vi "TRAJECTORY_CREATE_QUINTIC_BEGIN.vi"() -> (0 "Trajectory \ncalculation \nerror":errorcluster, 2 "Trajectory Items":i32, 3 "TotalTImeSecs":dbl)   [LabVIEW 2019]
uses:
  <vilib>/Rock Robotics/WPI/ThirdParty/JAS_Junk/TrajLib/Rotation_CreateAngle.vi
  <vilib>/Rock Robotics/WPI/ThirdParty/JAS_Junk/TrajLib/Translation_Create.vi
  <vilib>/Rock Robotics/SystemInterfaces/NetworkCommunication/NetComm_UsageReport_report.vi
  <vilib>/Rock Robotics/WPI/ThirdParty/JAS_Junk/TrajLib/DiffDriveKinematicsConstraint_New.vi
  <vilib>/Rock Robotics/WPI/ThirdParty/JAS_Junk/TrajLib/CentripetalAccelConstraint_New.vi
  <vilib>/Rock Robotics/WPI/ThirdParty/JAS_Junk/TrajLib/Util_LibraryGlobals.vi
  <vilib>/Rock Robotics/WPI/ThirdParty/JAS_Junk/TrajLib/Trajectory_Library.lvlib
panel:
  in  "WayPoints":T1(array[cluster])=[{"X Inches"=15.0, "Y Inches"=105.0, "Heading\nDegrees"=-45.0}, {"X Inches"=105.0, "Y Inches"=65.0, "Heading\nDegrees"=0.0}, {"X Inches"=210.0, "Y Inches"=105.0, "Heading\nDegrees"=45.0}]
  in  "Use Diff Drive\nKinematic\nConstraint":bool=TRUE
  in  "Use Centripetal\nAcceleration\nConstaint":bool=TRUE
  out "Wheelbase Width":dbl=0.66 format="%20.4f"
  out "MaxAcceleration":dbl=1.3 format="%17.4f"
  out "MaxVelocity":dbl=2.0 format="%17.4f"
  out "Max Cent Accel":dbl=1.0 format="%20.4f"
  in  "Max Cent Accel INCHES/SEC^2":dbl=15.0 format="%20.1f"
  in  "MaxAcceleration INCHES/SEC^2":dbl=30.0 format="%17.1f"
  in  "MaxVelocity Fraction":dbl=0.666 format="%17.3f"
  # "TRAJECTORY CONFIGURATION"
  # "20.9 real"
  # "TRAJECTORY DEFINITION"
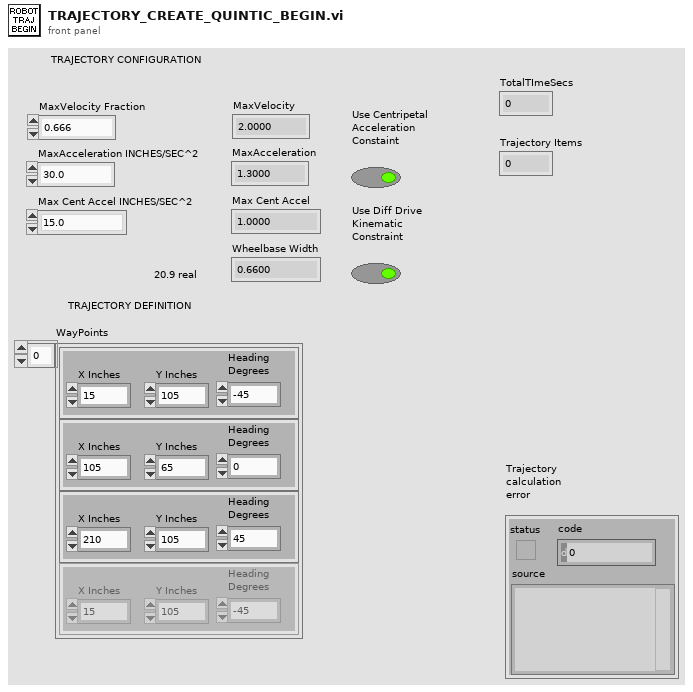
[diagram p1: front panel]
types:
  T1 = cluster{"X Inches":dbl, "Y Inches":dbl, "Heading\nDegrees":dbl}[]
  T2 = typedef "Trajectory_Library.lvlib/POSE2D.ctl" = cluster{"TRANSLATION":T3, "ROTATION":T4}
  T3 = typedef "Trajectory_Library.lvlib/TRANSLATION2D.ctl" = cluster{"X":dbl, "Y":dbl}
  T4 = typedef "Trajectory_Library.lvlib/ROTATION2D.ctl" = cluster{"VALUE":dbl, "COS":dbl, "SIN":dbl}
  T5 = typedef "Trajectory_Library.lvlib/TRAJ_CONFIG.ctl" = cluster{"MaxVelocity":dbl, "Max Acceleration":dbl, "StartVelocity":dbl, "End Velocity":dbl, "Reversed":bool, "DiffDrKineConstntDefined":bool, "CentAcellConstntDefined":bool, "DiffDrVoltConstntDefined":bool, "DIFF_DRIVE_KINE_CONSTRAINT":T6, "CENTRIPETAL_ACCEL_CONSTRAINT":T8, "SwerveDrKineConstntDefined":bool, "SWERVE_DRIVE_KINE_CONSTRAINT":T9, "DIFF_DRIVE_VOLTAGE_CONSTRAINT":T12, "MECANUM_DRIVE_KINE_CONSTRAINT":T14, "MecanumDrKineConstntDefined":bool}
  T6 = typedef "Trajectory_Library.lvlib/TRAJ_CONSTRAINT_DIIF_DRIVE_KINEMATICS.ctl" = cluster{"Max Speed (M/S)":dbl, "DIFF_DRIVE_KINEMATICS":T7}
  T7 = typedef "Trajectory_Library.lvlib/DIFF_DRIVE_KINEMATICS.ctl" = cluster{"TrackWidth_Meters":dbl}
  T8 = typedef "Trajectory_Library.lvlib/TRAJ_CONSTRAINT_CENTRIPETAL_ACCEL.ctl" = cluster{"Max Cent Accel":dbl}
  T9 = typedef "Trajectory_Library.lvlib/TRAJ_CONSTRAINT_SWERVE_DRIVE_KINEMATICS.ctl" = cluster{"Max Speed (M/S)":dbl, "SwerveKinematics":T10}
  T10 = typedef "Trajectory_Library.lvlib/SWERVE_DRIVE_KINEMATICS.ctl" = cluster{"NumModules":i32, "InverseKinematics":T11, "ForwardKinematics":T11, "Modules":T3[], "PrevCoR":T3}
  T11 = typedef "NI_Matrix.lvlib/RealMatrix.ctl" = dbl[][]
  T12 = typedef "Trajectory_Library.lvlib/TRAJ_CONSTRAINT_DIIF_DRIVE_VOLTAGE.ctl" = cluster{"Max Voltage":dbl, "DIFF_DRIVE_KINEMATICS":T7, "SIMPLE_MOTOR_FF":T13}
  T13 = typedef "Trajectory_Library.lvlib/SIMPLE_MOTOR_FF.ctl" = cluster{"Ks":dbl, "Kv":dbl, "Ka":dbl}
  T14 = typedef "Trajectory_Library.lvlib/TRAJ_CONSTRAINT_MECA_DRIVE_KINEMATICS.ctl" = cluster{"Max Speed (M/S)":dbl, "MECA_DRIVE_KINEMATICS":T15}
  T15 = typedef "Trajectory_Library.lvlib/MECA_DRIVE_KINEMATICS.ctl" = cluster{"FrontLeft":T3, "FrontRight":T3, "RearLeft":T3, "RearRight":T3, "InverseKinematics":T11, "ForwardKinematics":T11, "PrevCoR":T3}
  T16 = typedef "Trajectory_Library.lvlib/TRAJECTORY.ctl" = cluster{"TotalTImeSecs":dbl, "States":T17[]}
  T17 = typedef "Trajectory_Library.lvlib/TRAJ_STATE.ctl" = cluster{"TimeSeconds":dbl, "Velocity":dbl, "Acceleration":dbl, "POSE":T2, "Curvature":dbl}
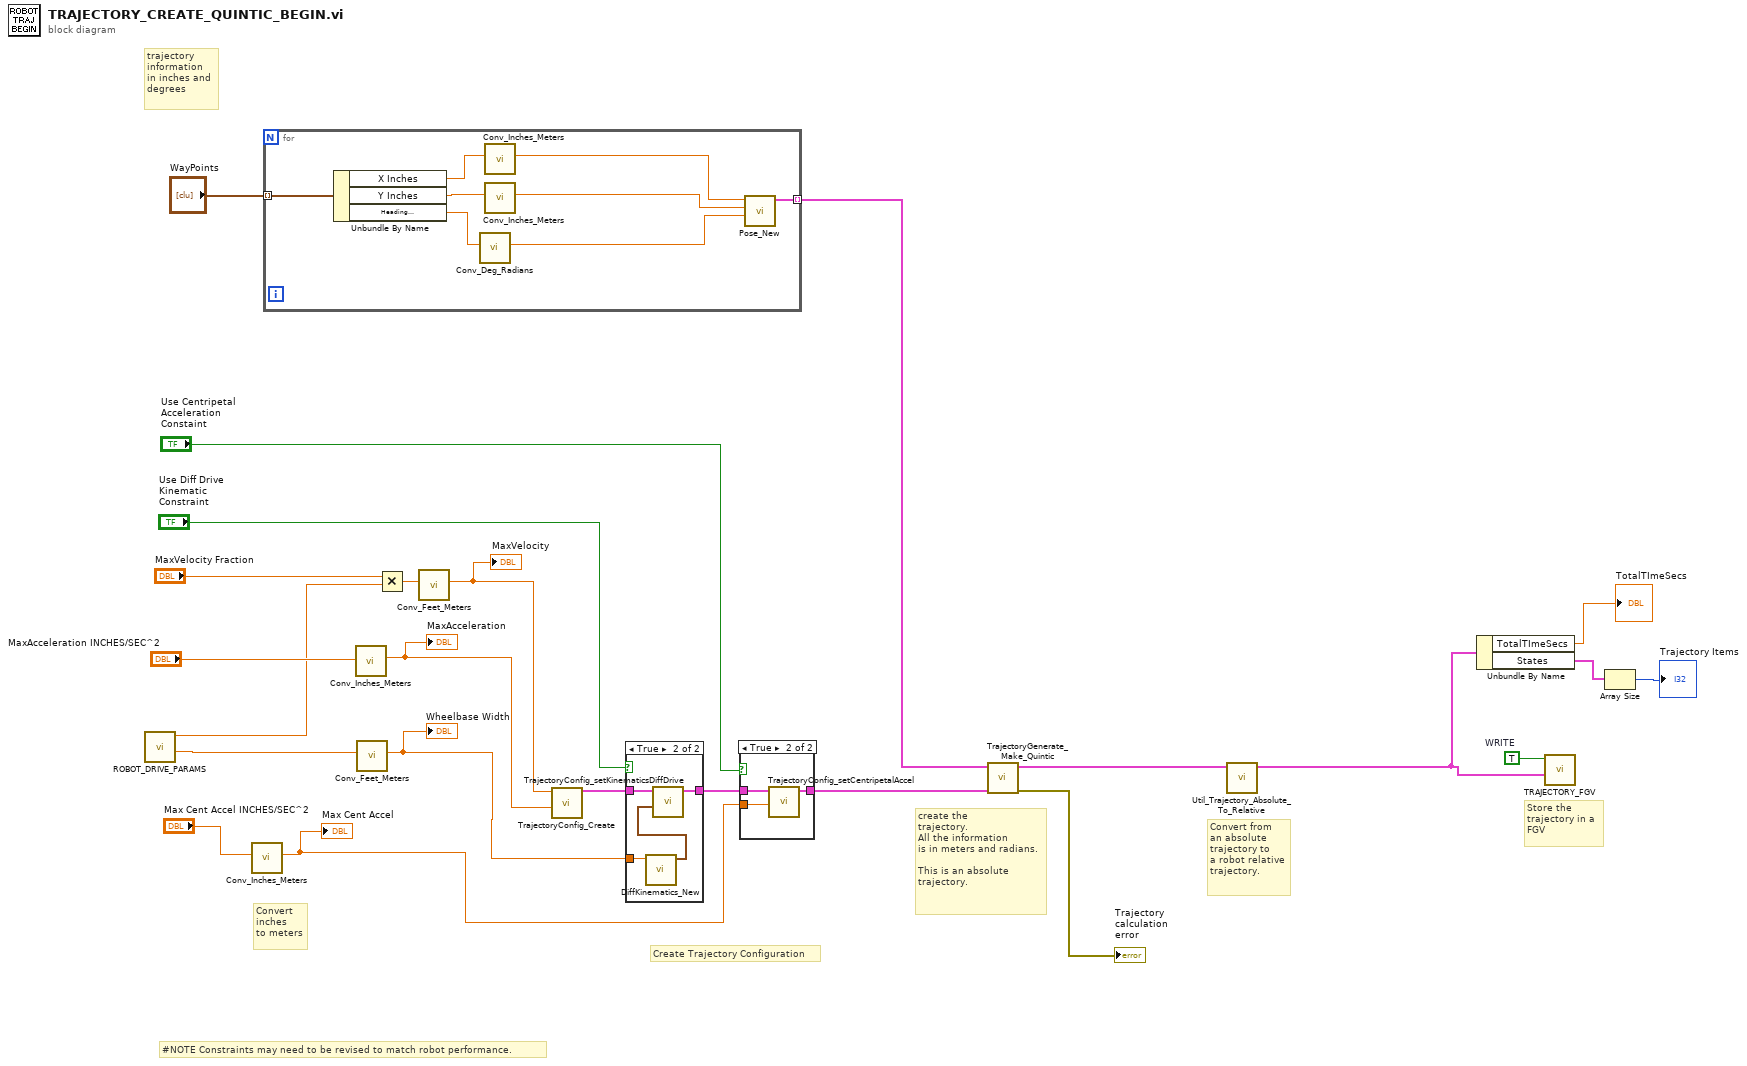
[diagram p0: block diagram]
diagram:
  w12 = TRUE  # WRITE
  # "#NOTE Constraints may need to be revised to match robot performance."
  # "Store the\ntrajectory in a \nFGV"
  # "Convert from\nan absolute\ntrajectory to\na robot relative\ntrajectory."
  # "Convert\ninches\nto meters"
  # "create the\ntrajectory.\nAll the information\nis in meters and radians.\n\nThis is an absolute \ntrajectory."
  # "trajectory\ninformation\nin inches and\ndegrees"
  # "Create Trajectory Configuration"
  n1 = call "ROBOT_DRIVE_PARAMS.vi"() -> ("Effective Wheelbase Ft"=w4:dbl, "Max Speed Ft/Sec"=w2:dbl)  [unwired: 10 in]
  n2 = call <vilib>:"Conv_Inches_Meters.vi"("INCH"="Max Cent Accel INCHES/SEC^2") -> ("Meters"=w17:dbl)  [unwired: 10 in]
  "Max Cent Accel" <- w17
  n3 = for {
    tunnel: [w30] -> w8 mode=indexing
    tunnel: "WayPoints" -> [w29] mode=indexing
    n4 = Unbundle By Name(w29) -> ("X Inches"=w32:dbl, "Y Inches"=w31:dbl, "Heading\nDegrees"=w26:dbl)
    n5 = call <vilib>:"Conv_Deg_Radians.vi"("Degress"=w26) -> ("Radians"=w25:dbl)  [unwired: 10 in]
    n6 = call <vilib>:"Conv_Inches_Meters.vi"("INCH"=w32) -> ("Meters"=w28:dbl)  [unwired: 10 in]
    n7 = call <vilib>:"Conv_Inches_Meters.vi"("INCH"=w31) -> ("Meters"=w27:dbl)  [unwired: 10 in]
    n8 = call <vilib>:"Pose_New.vi"("Heading"=w25, "Y"=w27, "X"=w28) -> ("out POSe"=w30:T2)  [unwired: 8 in]
  }
  n9 = call <vilib>:"Conv_Inches_Meters.vi"("INCH"="MaxAcceleration INCHES/SEC^2") -> ("Meters"=w16:dbl)  [unwired: 10 in]
  "MaxAcceleration" <- w16
  n10 = call <vilib>:"Conv_Feet_Meters.vi"("Feet"=w4) -> ("Meters"=w18:dbl)  [unwired: 10 in]
  "Wheelbase Width" <- w18
  n11 = Multiply(x="MaxVelocity Fraction", y=w2) -> (x*y=w3:dbl)
  n12 = call <vilib>:"Conv_Feet_Meters.vi"("Feet"=w3) -> ("Meters"=w15:dbl)  [unwired: 10 in]
  "MaxVelocity" <- w15
  n13 = call <vilib>:"TrajectoryConfig_Create.vi"("MaxAcceleration"=w16, "MaxVelocity"=w15) -> ("TRAJECTORY_CONFIG"=w22:T5)  [unwired: 9 in]
  n14 = case shown="True" "Use Diff Drive\nKinematic\nConstraint" {
    tunnel: w22 -> [w33 w37]
    tunnel: [w33 w36] -> w21
    tunnel: w18 -> [_ w34]
    frame False {
    }
    frame True {
      n15 = call <vilib>:"DiffKinematics_New.vi"("TrackWidth_Meters"=w34) -> ("DIFF_DRIVE_KINEMATICS"=w35:T7)  [unwired: 10 in]
      n16 = call <vilib>:"TrajectoryConfig_setKinematicsDiffDrive.vi"("DIFF_DRIVE_KINEMATICS"=w35, "inTRAJECTORY_CONFIG"=w37) -> ("outTRAJECTORY_CONFIG"=w36:T5)  [unwired: 9 in]
    }
  }
  n17 = case shown="True" "Use Centripetal\nAcceleration\nConstaint" {
    tunnel: w21 -> [w38 w41]
    tunnel: [w38 w40] -> w13
    tunnel: w17 -> [_ w39]
    frame False {
    }
    frame True {
      n18 = call <vilib>:"TrajectoryConfig_setCentripetalAccel.vi"("Max Cent Accel"=w39, "inTRAJECTORY_CONFIG"=w41) -> ("outTRAJECTORY_CONFIG"=w40:T5)  [unwired: 9 in]
    }
  }
  n19 = call <vilib>:"TrajectoryGenerate_Make_Quintic.vi"("traj_config"=w13, "waypointPOSE"=w8) -> ("error out"=→"Trajectory \ncalculation \nerror":errorcluster, "TRAJECTORY"=w6:T16)  [unwired: 8 in]
  n20 = call <vilib>:"Util_Trajectory_Absolute_To_Relative.vi"("absTRAJECTORY"=w6) -> ("outputRelativeTRAJECTORY"=w5:T16)  [unwired: 10 in]
  n21 = Unbundle By Name(w5) -> ("TotalTImeSecs"=→"TotalTImeSecs":dbl, "States"=w10:T17[])
  n22 = call "TRAJECTORY_FGV.vi"("inTRAJECTORY"=w5, "WRITE"=w12) -> ()  [unwired: 9 in, 1 out]
  n23 = Array Size(array=w10) -> (size(s)=→"Trajectory Items":i32)
